vi "ADAM -12.vi"() -> ()   [LabVIEW 2016]
uses:
  <vilib>/Instr/_visa.llb/VISA Configure Serial Port (Instr).vi
panel:
  out "I 7_3":string
  out "I 6_3":string
  out "I 5_3":string
  out "I 4_3":string
  out "I 3_3":string
  out "I 2_3":string
  out "I 7_2":string
  out "I 6_2":string
  out "I 5_2":string
  out "I 4_2":string
  out "I 3_2":string
  out "I 2_2":string
  out "I 1_2":string
  out "I 0_2":string
  out "I 7_1":string
  out "I 6_1":string
  out "I 5_1":string
  out "I 4_1":string
  out "I 3_1":string
  out "I 2_1":string
  out "I 1_1":string
  out "I 0_1":string
  out "I 1_3":string
  out "I 0_3":string
  in  "rele 1_6":bool
  in  "rele 7_6":bool
  in  "rele 6_6":bool
  in  "rele 5_6":bool
  in  "rele 4_6":bool
  in  "rele 3_6":bool
  in  "rele 2_6":bool
  in  "rele 0_6":bool
  in  "rele 1_5":bool
  in  "rele 7_5":bool
  in  "rele 6_5":bool
  in  "rele 5_5":bool
  in  "rele 4_5":bool
  in  "rele 3_5":bool
  in  "rele 2_5":bool
  in  "rele 0_5":bool
  out "read buffer 3":string
  out "5_3":bool
  out "4_3":bool
  out "3_3":bool
  out "2_3":bool
  out "1_3":bool
  out "0_3":bool
  out "6_3":bool
  out "7_3":bool
  out "read buffer 2":string
  out "5_2":bool
  out "4_2":bool
  out "3_2":bool
  out "2_2":bool
  out "1_2":bool
  out "0_2":bool
  out "6_2":bool
  out "7_2":bool
  out "7_1":bool
  out "6_1":bool
  out "0_1":bool
  out "1_1":bool
  out "2_1":bool
  out "3_1":bool
  out "4_1":bool
  out "5_1":bool
  out "read buffer":string
  in  "all rele":bool
  in  "rele 1_4":bool
  in  "rele 7_4":bool
  in  "rele 6_4":bool
  in  "rele 5_4":bool
  in  "rele 4_4":bool
  in  "rele 3_4":bool
  in  "rele 2_4":bool
  in  "VISA rele":refnum<visa-resource-name>
  in  "rele 0_4":bool
  in  "stop":bool
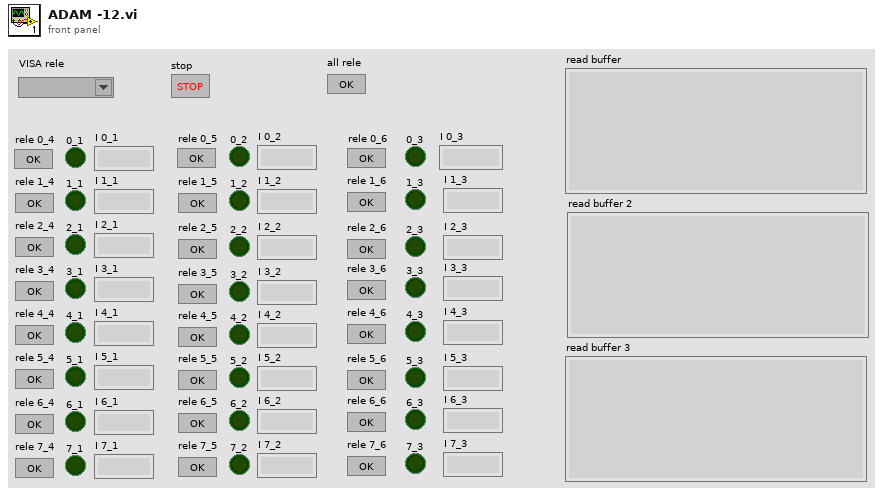
[diagram p1: front panel]
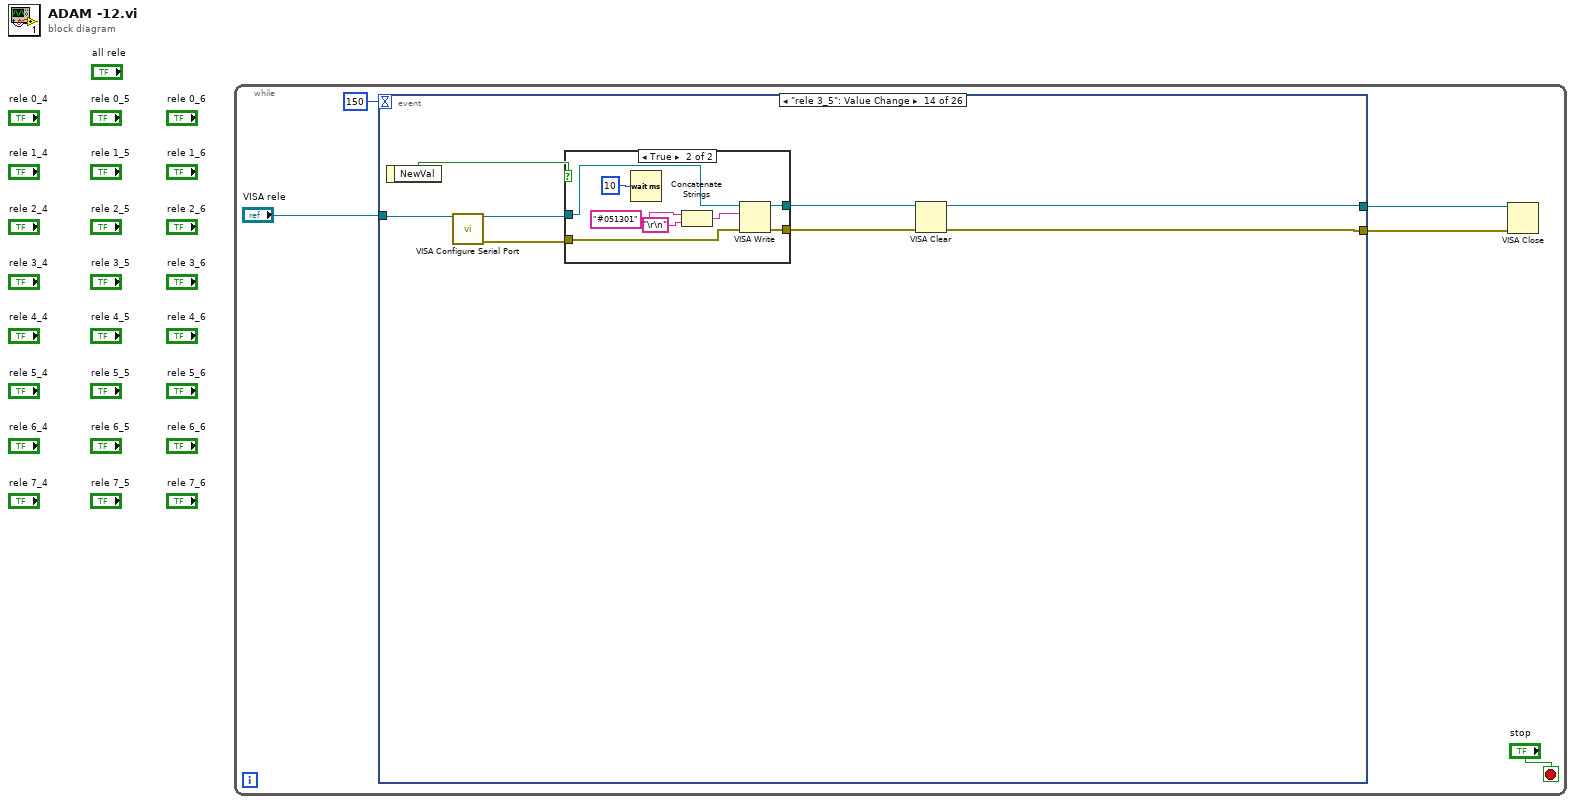
[diagram p0: block diagram]
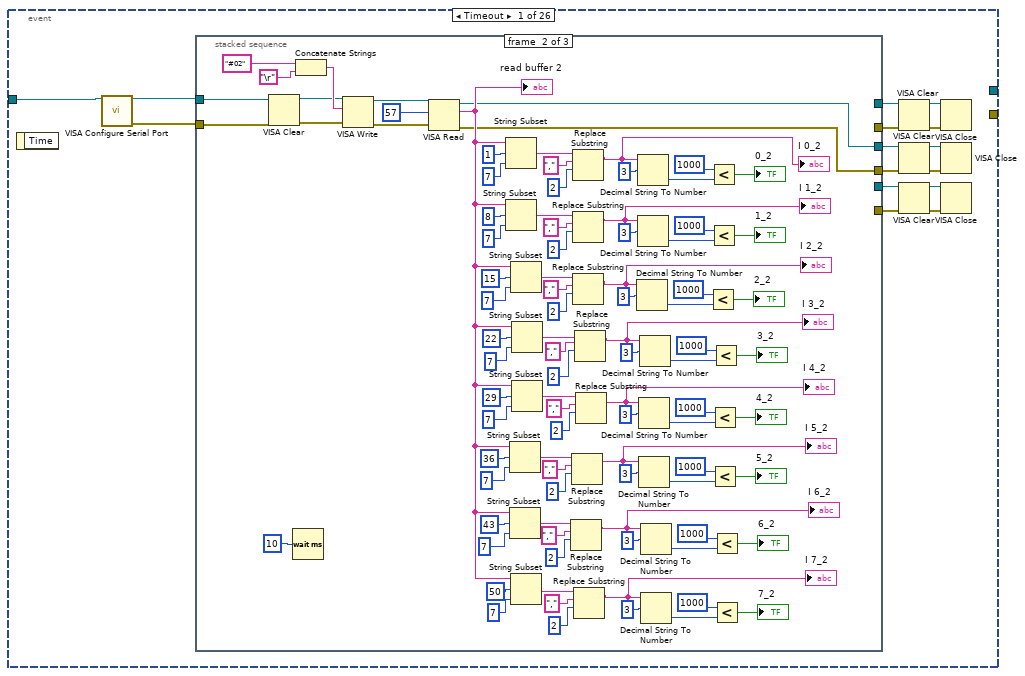
[diagram p2: hidden frame]
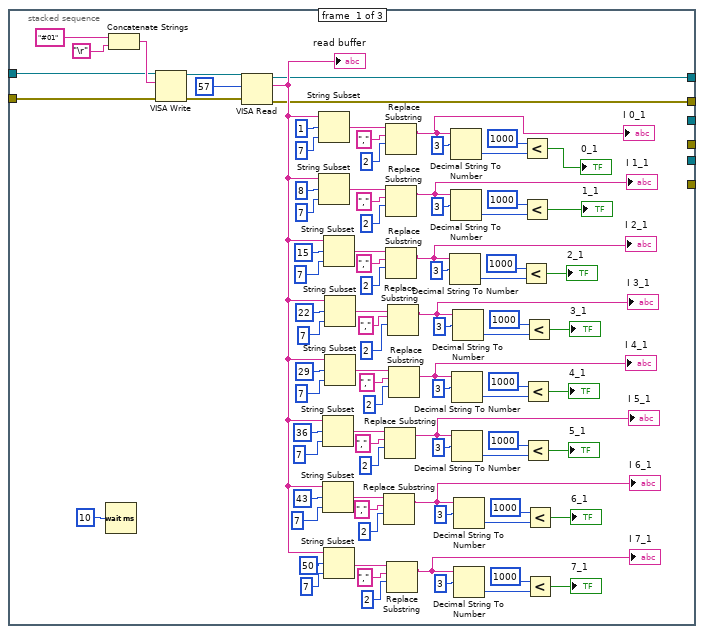
[diagram p3: hidden frame]
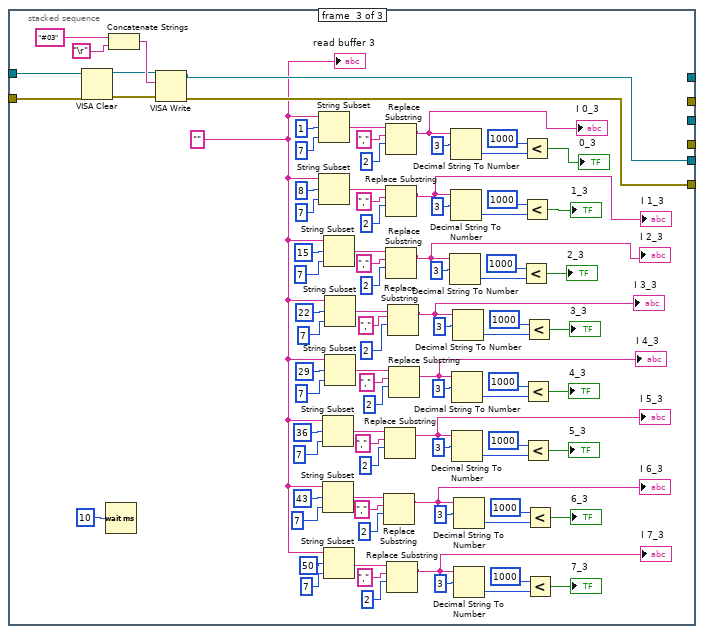
[diagram p4: hidden frame]
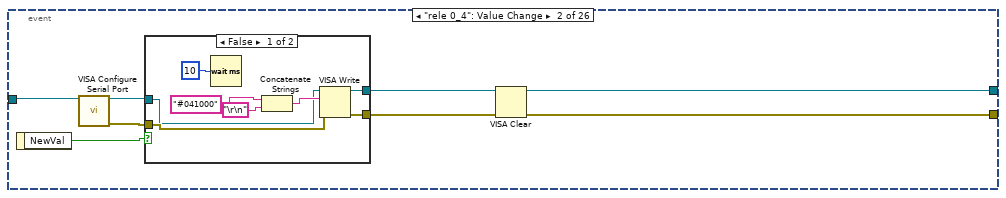
[diagram p5: hidden frame]
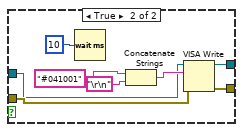
[diagram p6: hidden frame]
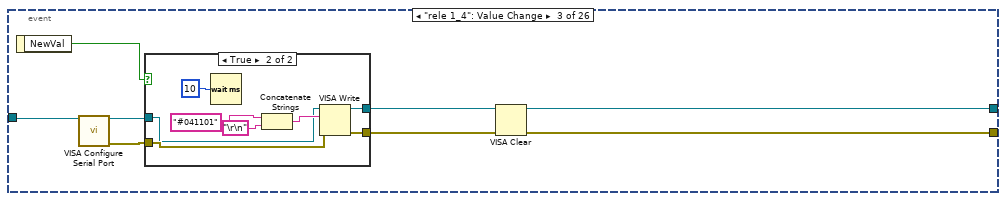
[diagram p7: hidden frame]
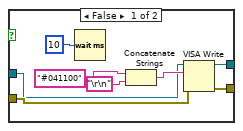
[diagram p8: hidden frame]
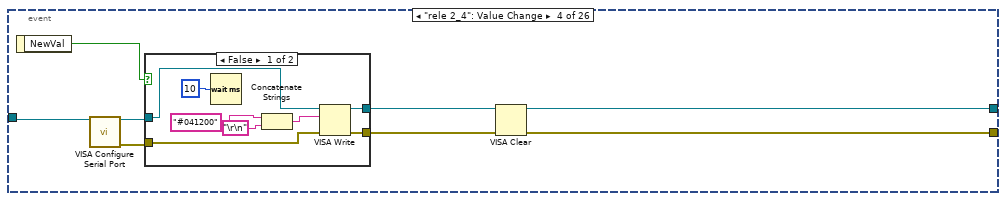
[diagram p9: hidden frame]
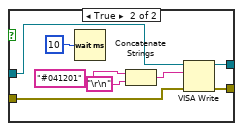
[diagram p10: hidden frame]
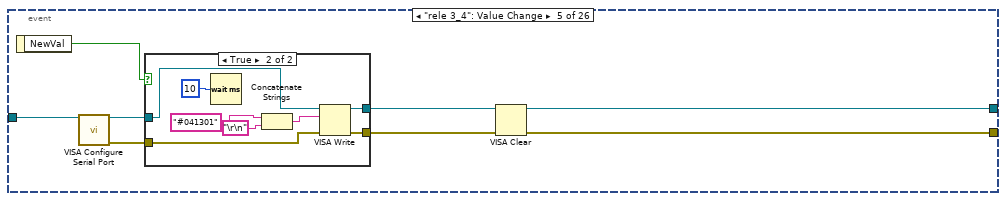
[diagram p11: hidden frame]
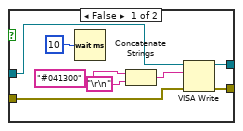
[diagram p12: hidden frame]
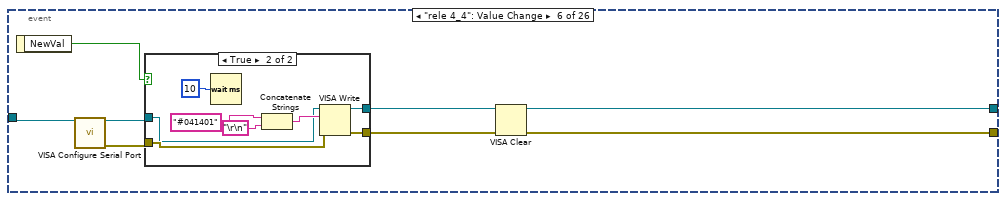
[diagram p13: hidden frame]
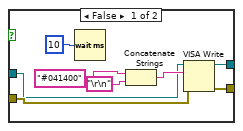
[diagram p14: hidden frame]
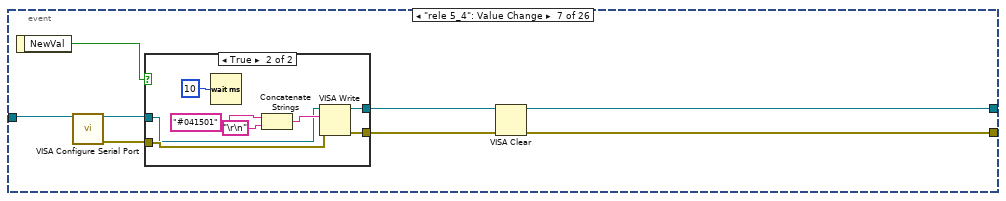
[diagram p15: hidden frame]
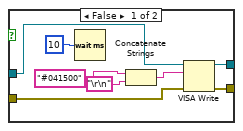
[diagram p16: hidden frame]
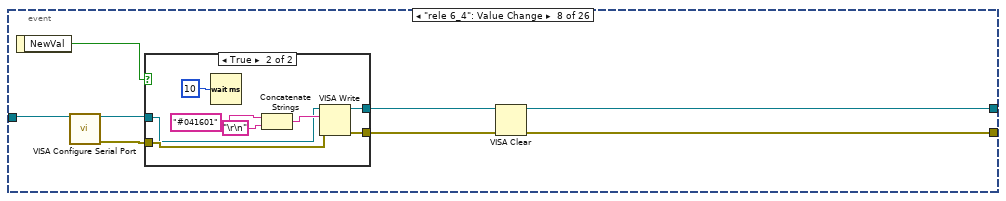
[diagram p17: hidden frame]
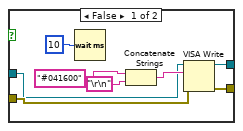
[diagram p18: hidden frame]
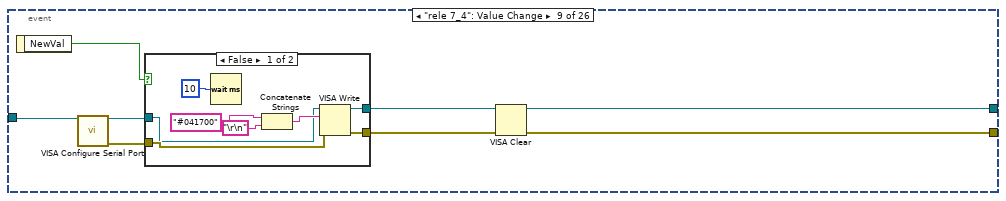
[diagram p19: hidden frame]
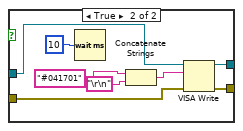
[diagram p20: hidden frame]
diagram:
  n1 = while {
    stop <- "stop" stop-if-true
    n2 = event shown="[13] \"rele 3_5\": Value Change" {
      selector: _ -> [_ _ _ _ _ _ _ _ _ _ _ _ _ _ _ _ _ _ _ _ _ _ _ _ _ _]
      dyn-events: _ -> [_ _ _ _ _ _ _ _ _ _ _ _ _ _ _ _ _ _ _ _ _ _ _ _ _ _]
      timeout: 150 -> [_ _ _ _ _ _ _ _ _ _ _ _ _ _ _ _ _ _ _ _ _ _ _ _ _ _]
      tunnel: "VISA rele" -> [w6 w298 w322 w346 w370 w394 w418 w442 w466 w490 w594 w618 w642 w666 w690 w714 w738 w762 w788 w810 w835 w858 w882 w906 w930 w954]
      tunnel: [_ w302 w326 w350 w374 w398 w422 w446 w470 w494 w598 w621 w646 w670 w694 w719 w742 w766 w790 w814 w838 w862 w886 w910 w934 w958] -> w3
      tunnel: [_ w301 w325 w349 w373 w397 w421 w445 w469 w493 w597 w622 w645 w669 w693 w718 w741 w765 w789 w813 w837 w861 w885 w909 w933 w957] -> w2
      event Timeout {
        n3 = event-data() -> ()  [unwired: 1 in, 1 out]
        n4 = call-poly "VISA Configure Serial Port"("VISA resource name"=w6) -> ("VISA resource name out"=w8:refnum<visa-resource-name>, "error out"=w7:errorcluster)  [unwired: 13 in]
        n5 = stacked-sequence {
          tunnel: w7 -> [w109 w124 w222]
          tunnel: w8 -> [w108 w123 w221]
          tunnel: [w62 _ _] -> w20
          tunnel: [w61 _ _] -> w17
          tunnel: [_ w126 _] -> w14
          tunnel: [_ w125 _] -> w13
          tunnel: [_ _ w218] -> w10
          tunnel: [_ _ w217] -> w9
          frame #0 {
            n6 = Wait (ms)(milliseconds to wait=u32 10) -> ()  [unwired: 1 out]
            n7 = Concatenate Strings("#01" ("string"), "\r") -> (w112:string)
            n8 = VISA Write(VISA resource name=w108, write buffer=w112, error in (no error)=w109) -> (VISA resource name out=w66:refnum<visa-resource-name>, error out=w65:errorcluster)  [unwired: 1 out]
            n9 = VISA Read(VISA resource name=w66, byte count=u32 57, error in (no error)=w65) -> (VISA resource name out=w61:refnum<visa-resource-name>, read buffer=w67:string, error out=w62:errorcluster)  [unwired: 1 out]
            "read buffer" <- w67
            n10 = String Subset(string=w67, offset (0)=1, length (rest)=7 ("length (rest)")) -> (substring=w84:string)
            n11 = String Subset(string=w67, offset (0)=8, length (rest)=7 ("length (rest)")) -> (substring=w89:string)
            n12 = String Subset(string=w67, offset (0)=36, length (rest)=7 ("length (rest)")) -> (substring=w101:string)
            n13 = String Subset(string=w67, offset (0)=43, length (rest)=7 ("length (rest)")) -> (substring=w104:string)
            n14 = String Subset(string=w67, offset (0)=15, length (rest)=7 ("length (rest)")) -> (substring=w92:string)
            n15 = String Subset(string=w67, offset (0)=50, length (rest)=7 ("length (rest)")) -> (substring=w107:string)
            n16 = String Subset(string=w67, offset (0)=22, length (rest)=7 ("length (rest)")) -> (substring=w95:string)
            n17 = String Subset(string=w67, offset (0)=29, length (rest)=7 ("length (rest)")) -> (substring=w98:string)
            n18 = Replace Substring(3:2 ("offset (0)"), 4:"," ("substring (\"\")"), 5:w104) -> (1:w22:string)  [unwired: 1 in, 1 out]
            "I 6_1" <- w22
            n19 = Replace Substring(3:2 ("offset (0)"), 4:"," ("substring (\"\")"), 5:w101) -> (1:w23:string)  [unwired: 1 in, 1 out]
            "I 5_1" <- w23
            n20 = Replace Substring(3:2 ("offset (0)"), 4:"," ("substring (\"\")"), 5:w84) -> (1:w28:string)  [unwired: 1 in, 1 out]
            "I 0_1" <- w28
            n21 = Replace Substring(3:2 ("offset (0)"), 4:"," ("substring (\"\")"), 5:w89) -> (1:w27:string)  [unwired: 1 in, 1 out]
            "I 1_1" <- w27
            n22 = Replace Substring(3:2 ("offset (0)"), 4:"," ("substring (\"\")"), 5:w92) -> (1:w26:string)  [unwired: 1 in, 1 out]
            "I 2_1" <- w26
            n23 = Replace Substring(3:2 ("offset (0)"), 4:"," ("substring (\"\")"), 5:w107) -> (1:w21:string)  [unwired: 1 in, 1 out]
            "I 7_1" <- w21
            n24 = Replace Substring(3:2 ("offset (0)"), 4:"," ("substring (\"\")"), 5:w95) -> (1:w25:string)  [unwired: 1 in, 1 out]
            "I 3_1" <- w25
            n25 = Replace Substring(3:2 ("offset (0)"), 4:"," ("substring (\"\")"), 5:w98) -> (1:w24:string)  [unwired: 1 in, 1 out]
            "I 4_1" <- w24
            n26 = Decimal String To Number(string=w26, offset=3) -> (number=w47:i32)  [unwired: 1 in, 1 out]
            n27 = Decimal String To Number(string=w28, offset=3) -> (number=w39:i32)  [unwired: 1 in, 1 out]
            n28 = Decimal String To Number(string=w27, offset=3) -> (number=w43:i32)  [unwired: 1 in, 1 out]
            n29 = Decimal String To Number(string=w24, offset=3) -> (number=w55:i32)  [unwired: 1 in, 1 out]
            n30 = Decimal String To Number(string=w23, offset=3) -> (number=w59:i32)  [unwired: 1 in, 1 out]
            n31 = Decimal String To Number(string=w25, offset=3) -> (number=w51:i32)  [unwired: 1 in, 1 out]
            n32 = Decimal String To Number(string=w22, offset=3) -> (number=w35:i32)  [unwired: 1 in, 1 out]
            n33 = Decimal String To Number(string=w21, offset=3) -> (number=w31:i32)  [unwired: 1 in, 1 out]
            n34 = Less?(x=1000, y=w47) -> (x < y?=→"2_1":bool)
            n35 = Less?(x=1000, y=w39) -> (x < y?=→"0_1":bool)
            n36 = Less?(x=1000, y=w43) -> (x < y?=→"1_1":bool)
            n37 = Less?(x=1000, y=w55) -> (x < y?=→"4_1":bool)
            n38 = Less?(x=1000, y=w59) -> (x < y?=→"5_1":bool)
            n39 = Less?(x=1000, y=w51) -> (x < y?=→"3_1":bool)
            n40 = Less?(x=1000, y=w35) -> (x < y?=→"6_1":bool)
            n41 = Less?(x=1000, y=w31) -> (x < y?=→"7_1":bool)
          }
          frame #1 {
            n42 = VISA Clear(VISA resource name=w123, error in (no error)=w124) -> (VISA resource name out=w121:refnum<visa-resource-name>, error out=w122:errorcluster)
            n43 = Wait (ms)(milliseconds to wait=u32 10) -> ()  [unwired: 1 out]
            n44 = Concatenate Strings("#02" ("string"), "\r") -> (w206:string)
            n45 = VISA Write(VISA resource name=w121, write buffer=w206, error in (no error)=w122) -> (VISA resource name out=w162:refnum<visa-resource-name>, error out=w161:errorcluster)  [unwired: 1 out]
            n46 = VISA Read(VISA resource name=w162, byte count=u32 57, error in (no error)=w161) -> (VISA resource name out=w125:refnum<visa-resource-name>, read buffer=w163:string, error out=w126:errorcluster)  [unwired: 1 out]
            "read buffer 2" <- w163
            n47 = String Subset(string=w163, offset (0)=1, length (rest)=7 ("length (rest)")) -> (substring=w180:string)
            n48 = String Subset(string=w163, offset (0)=8, length (rest)=7 ("length (rest)")) -> (substring=w185:string)
            n49 = String Subset(string=w163, offset (0)=36, length (rest)=7 ("length (rest)")) -> (substring=w197:string)
            n50 = String Subset(string=w163, offset (0)=43, length (rest)=7 ("length (rest)")) -> (substring=w200:string)
            n51 = String Subset(string=w163, offset (0)=15, length (rest)=7 ("length (rest)")) -> (substring=w188:string)
            n52 = String Subset(string=w163, offset (0)=50, length (rest)=7 ("length (rest)")) -> (substring=w203:string)
            n53 = String Subset(string=w163, offset (0)=22, length (rest)=7 ("length (rest)")) -> (substring=w191:string)
            n54 = String Subset(string=w163, offset (0)=29, length (rest)=7 ("length (rest)")) -> (substring=w194:string)
            n55 = Replace Substring(3:2 ("offset (0)"), 4:"," ("substring (\"\")"), 5:w200) -> (1:w114:string)  [unwired: 1 in, 1 out]
            "I 6_2" <- w114
            n56 = Replace Substring(3:2 ("offset (0)"), 4:"," ("substring (\"\")"), 5:w197) -> (1:w115:string)  [unwired: 1 in, 1 out]
            "I 5_2" <- w115
            n57 = Replace Substring(3:2 ("offset (0)"), 4:"," ("substring (\"\")"), 5:w180) -> (1:w120:string)  [unwired: 1 in, 1 out]
            "I 0_2" <- w120
            n58 = Replace Substring(3:2 ("offset (0)"), 4:"," ("substring (\"\")"), 5:w185) -> (1:w119:string)  [unwired: 1 in, 1 out]
            "I 1_2" <- w119
            n59 = Replace Substring(3:2 ("offset (0)"), 4:"," ("substring (\"\")"), 5:w188) -> (1:w118:string)  [unwired: 1 in, 1 out]
            "I 2_2" <- w118
            n60 = Replace Substring(3:2 ("offset (0)"), 4:"," ("substring (\"\")"), 5:w203) -> (1:w113:string)  [unwired: 1 in, 1 out]
            "I 7_2" <- w113
            n61 = Replace Substring(3:2 ("offset (0)"), 4:"," ("substring (\"\")"), 5:w191) -> (1:w117:string)  [unwired: 1 in, 1 out]
            "I 3_2" <- w117
            n62 = Replace Substring(3:2 ("offset (0)"), 4:"," ("substring (\"\")"), 5:w194) -> (1:w116:string)  [unwired: 1 in, 1 out]
            "I 4_2" <- w116
            n63 = Decimal String To Number(string=w118, offset=3) -> (number=w145:i32)  [unwired: 1 in, 1 out]
            n64 = Decimal String To Number(string=w120, offset=3) -> (number=w137:i32)  [unwired: 1 in, 1 out]
            n65 = Decimal String To Number(string=w119, offset=3) -> (number=w141:i32)  [unwired: 1 in, 1 out]
            n66 = Decimal String To Number(string=w116, offset=3) -> (number=w153:i32)  [unwired: 1 in, 1 out]
            n67 = Decimal String To Number(string=w115, offset=3) -> (number=w157:i32)  [unwired: 1 in, 1 out]
            n68 = Decimal String To Number(string=w117, offset=3) -> (number=w149:i32)  [unwired: 1 in, 1 out]
            n69 = Decimal String To Number(string=w114, offset=3) -> (number=w133:i32)  [unwired: 1 in, 1 out]
            n70 = Decimal String To Number(string=w113, offset=3) -> (number=w129:i32)  [unwired: 1 in, 1 out]
            n71 = Less?(x=1000, y=w145) -> (x < y?=→"2_2":bool)
            n72 = Less?(x=1000, y=w137) -> (x < y?=→"0_2":bool)
            n73 = Less?(x=1000, y=w141) -> (x < y?=→"1_2":bool)
            n74 = Less?(x=1000, y=w153) -> (x < y?=→"4_2":bool)
            n75 = Less?(x=1000, y=w157) -> (x < y?=→"5_2":bool)
            n76 = Less?(x=1000, y=w149) -> (x < y?=→"3_2":bool)
            n77 = Less?(x=1000, y=w133) -> (x < y?=→"6_2":bool)
            n78 = Less?(x=1000, y=w129) -> (x < y?=→"7_2":bool)
          }
          frame #2 {
            w216 = "" ("string")
            n79 = VISA Clear(VISA resource name=w221, error in (no error)=w222) -> (VISA resource name out=w219:refnum<visa-resource-name>, error out=w220:errorcluster)
            n80 = Wait (ms)(milliseconds to wait=u32 10) -> ()  [unwired: 1 out]
            n81 = Concatenate Strings("#03" ("string"), "\r") -> (w297:string)
            n82 = VISA Write(VISA resource name=w219, write buffer=w297, error in (no error)=w220) -> (VISA resource name out=w218:refnum<visa-resource-name>, error out=w217:errorcluster)  [unwired: 1 out]
            n83 = String Subset(string=w216, offset (0)=1, length (rest)=7 ("length (rest)")) -> (substring=w214:string)
            n84 = String Subset(string=w216, offset (0)=8, length (rest)=7 ("length (rest)")) -> (substring=w276:string)
            n85 = String Subset(string=w216, offset (0)=36, length (rest)=7 ("length (rest)")) -> (substring=w288:string)
            n86 = String Subset(string=w216, offset (0)=43, length (rest)=7 ("length (rest)")) -> (substring=w291:string)
            n87 = String Subset(string=w216, offset (0)=15, length (rest)=7 ("length (rest)")) -> (substring=w279:string)
            n88 = String Subset(string=w216, offset (0)=50, length (rest)=7 ("length (rest)")) -> (substring=w294:string)
            n89 = String Subset(string=w216, offset (0)=22, length (rest)=7 ("length (rest)")) -> (substring=w282:string)
            n90 = String Subset(string=w216, offset (0)=29, length (rest)=7 ("length (rest)")) -> (substring=w285:string)
            n91 = Replace Substring(3:2 ("offset (0)"), 4:"," ("substring (\"\")"), 5:w291) -> (1:w208:string)  [unwired: 1 in, 1 out]
            "I 6_3" <- w208
            n92 = Replace Substring(3:2 ("offset (0)"), 4:"," ("substring (\"\")"), 5:w288) -> (1:w209:string)  [unwired: 1 in, 1 out]
            "I 5_3" <- w209
            n93 = Replace Substring(3:2 ("offset (0)"), 4:"," ("substring (\"\")"), 5:w214) -> (1:w213:string)  [unwired: 1 in, 1 out]
            "I 0_3" <- w213
            n94 = Replace Substring(3:2 ("offset (0)"), 4:"," ("substring (\"\")"), 5:w276) -> (1:w215:string)  [unwired: 1 in, 1 out]
            "I 1_3" <- w215
            n95 = Replace Substring(3:2 ("offset (0)"), 4:"," ("substring (\"\")"), 5:w279) -> (1:w212:string)  [unwired: 1 in, 1 out]
            "I 2_3" <- w212
            n96 = Replace Substring(3:2 ("offset (0)"), 4:"," ("substring (\"\")"), 5:w294) -> (1:w207:string)  [unwired: 1 in, 1 out]
            "I 7_3" <- w207
            n97 = Replace Substring(3:2 ("offset (0)"), 4:"," ("substring (\"\")"), 5:w282) -> (1:w211:string)  [unwired: 1 in, 1 out]
            "I 3_3" <- w211
            n98 = Replace Substring(3:2 ("offset (0)"), 4:"," ("substring (\"\")"), 5:w285) -> (1:w210:string)  [unwired: 1 in, 1 out]
            "I 4_3" <- w210
            n99 = Decimal String To Number(string=w212, offset=3) -> (number=w241:i32)  [unwired: 1 in, 1 out]
            n100 = Decimal String To Number(string=w213, offset=3) -> (number=w233:i32)  [unwired: 1 in, 1 out]
            n101 = Decimal String To Number(string=w215, offset=3) -> (number=w237:i32)  [unwired: 1 in, 1 out]
            n102 = Decimal String To Number(string=w210, offset=3) -> (number=w249:i32)  [unwired: 1 in, 1 out]
            n103 = Decimal String To Number(string=w209, offset=3) -> (number=w253:i32)  [unwired: 1 in, 1 out]
            n104 = Decimal String To Number(string=w211, offset=3) -> (number=w245:i32)  [unwired: 1 in, 1 out]
            n105 = Decimal String To Number(string=w208, offset=3) -> (number=w229:i32)  [unwired: 1 in, 1 out]
            n106 = Decimal String To Number(string=w207, offset=3) -> (number=w225:i32)  [unwired: 1 in, 1 out]
            n107 = Less?(x=1000, y=w241) -> (x < y?=→"2_3":bool)
            n108 = Less?(x=1000, y=w233) -> (x < y?=→"0_3":bool)
            n109 = Less?(x=1000, y=w237) -> (x < y?=→"1_3":bool)
            n110 = Less?(x=1000, y=w249) -> (x < y?=→"4_3":bool)
            n111 = Less?(x=1000, y=w253) -> (x < y?=→"5_3":bool)
            n112 = Less?(x=1000, y=w245) -> (x < y?=→"3_3":bool)
            n113 = Less?(x=1000, y=w229) -> (x < y?=→"6_3":bool)
            n114 = Less?(x=1000, y=w225) -> (x < y?=→"7_3":bool)
            "read buffer 3" <- w216
          }
        }
        n115 = VISA Clear(VISA resource name=w17, error in (no error)=w20) -> (VISA resource name out=w15:refnum<visa-resource-name>, error out=w16:errorcluster)
        n116 = VISA Clear(VISA resource name=w13, error in (no error)=w14) -> (VISA resource name out=w19:refnum<visa-resource-name>, error out=w18:errorcluster)
        n117 = VISA Clear(VISA resource name=w10, error in (no error)=w9) -> (VISA resource name out=w12:refnum<visa-resource-name>, error out=w11:errorcluster)
        n118 = VISA Close(VISA resource name=w15, error in (no error)=w16) -> ()  [unwired: 1 out]
        n119 = VISA Close(VISA resource name=w19, error in (no error)=w18) -> ()  [unwired: 1 out]
        n120 = VISA Close(VISA resource name=w12, error in (no error)=w11) -> ()  [unwired: 1 out]
      }
      event "rele 0_4": Value Change {
        n121 = event-data() -> ("NewVal"=w305:bool)  [unwired: 1 in]
        n122 = call-poly "VISA Configure Serial Port"("VISA resource name"=w298) -> ("VISA resource name out"=w299:refnum<visa-resource-name>, "error out"=w300:errorcluster)  [unwired: 13 in]
        n123 = case shown="False" w305 {
          tunnel: [w310 w318] -> w303
          tunnel: [w309 w317] -> w304
          tunnel: w300 -> [w308 w316]
          tunnel: w299 -> [w307 w315]
          frame False {
            n124 = Wait (ms)(milliseconds to wait=u32 10) -> ()  [unwired: 1 out]
            n125 = Concatenate Strings("#041000" ("string"), "\r\n") -> (w313:string)
            n126 = VISA Write(VISA resource name=w307, write buffer=w313, error in (no error)=w308) -> (VISA resource name out=w310:refnum<visa-resource-name>, error out=w309:errorcluster)  [unwired: 1 out]
          }
          frame True {
            n127 = Wait (ms)(milliseconds to wait=u32 10) -> ()  [unwired: 1 out]
            n128 = Concatenate Strings("#041001" ("string"), "\r\n") -> (w321:string)
            n129 = VISA Write(VISA resource name=w315, write buffer=w321, error in (no error)=w316) -> (VISA resource name out=w318:refnum<visa-resource-name>, error out=w317:errorcluster)  [unwired: 1 out]
          }
        }
        n130 = VISA Clear(VISA resource name=w303, error in (no error)=w304) -> (VISA resource name out=w301:refnum<visa-resource-name>, error out=w302:errorcluster)
      }
      event "rele 1_4": Value Change {
        n131 = event-data() -> ("NewVal"=w329:bool)  [unwired: 1 in]
        n132 = call-poly "VISA Configure Serial Port"("VISA resource name"=w322) -> ("VISA resource name out"=w324:refnum<visa-resource-name>, "error out"=w323:errorcluster)  [unwired: 13 in]
        n133 = case shown="True" w329 {
          tunnel: [w334 w342] -> w328
          tunnel: [w333 w341] -> w327
          tunnel: w323 -> [w331 w339]
          tunnel: w324 -> [w330 w338]
          frame False {
            n134 = Wait (ms)(milliseconds to wait=u32 10) -> ()  [unwired: 1 out]
            n135 = Concatenate Strings("#041100" ("string"), "\r\n") -> (w337:string)
            n136 = VISA Write(VISA resource name=w330, write buffer=w337, error in (no error)=w331) -> (VISA resource name out=w333:refnum<visa-resource-name>, error out=w334:errorcluster)  [unwired: 1 out]
          }
          frame True {
            n137 = Wait (ms)(milliseconds to wait=u32 10) -> ()  [unwired: 1 out]
            n138 = Concatenate Strings("#041101" ("string"), "\r\n") -> (w345:string)
            n139 = VISA Write(VISA resource name=w338, write buffer=w345, error in (no error)=w339) -> (VISA resource name out=w341:refnum<visa-resource-name>, error out=w342:errorcluster)  [unwired: 1 out]
          }
        }
        n140 = VISA Clear(VISA resource name=w327, error in (no error)=w328) -> (VISA resource name out=w325:refnum<visa-resource-name>, error out=w326:errorcluster)
      }
      event "rele 2_4": Value Change {
        n141 = event-data() -> ("NewVal"=w353:bool)  [unwired: 1 in]
        n142 = call-poly "VISA Configure Serial Port"("VISA resource name"=w346) -> ("VISA resource name out"=w348:refnum<visa-resource-name>, "error out"=w347:errorcluster)  [unwired: 13 in]
        n143 = case shown="False" w353 {
          tunnel: [w356 w366] -> w352
          tunnel: [w355 w365] -> w351
          tunnel: w348 -> [w358 w364]
          tunnel: w347 -> [w357 w363]
          frame False {
            n144 = Wait (ms)(milliseconds to wait=u32 10) -> ()  [unwired: 1 out]
            n145 = Concatenate Strings("#041200" ("string"), "\r\n") -> (w361:string)
            n146 = VISA Write(VISA resource name=w358, write buffer=w361, error in (no error)=w357) -> (VISA resource name out=w355:refnum<visa-resource-name>, error out=w356:errorcluster)  [unwired: 1 out]
          }
          frame True {
            n147 = Wait (ms)(milliseconds to wait=u32 10) -> ()  [unwired: 1 out]
            n148 = Concatenate Strings("#041201" ("string"), "\r\n") -> (w369:string)
            n149 = VISA Write(VISA resource name=w364, write buffer=w369, error in (no error)=w363) -> (VISA resource name out=w365:refnum<visa-resource-name>, error out=w366:errorcluster)  [unwired: 1 out]
          }
        }
        n150 = VISA Clear(VISA resource name=w351, error in (no error)=w352) -> (VISA resource name out=w349:refnum<visa-resource-name>, error out=w350:errorcluster)
      }
      event "rele 3_4": Value Change {
        n151 = event-data() -> ("NewVal"=w377:bool)  [unwired: 1 in]
        n152 = call-poly "VISA Configure Serial Port"("VISA resource name"=w370) -> ("VISA resource name out"=w372:refnum<visa-resource-name>, "error out"=w371:errorcluster)  [unwired: 13 in]
        n153 = case shown="True" w377 {
          tunnel: w372 -> [w382 w390]
          tunnel: w371 -> [w381 w389]
          tunnel: [w380 w387] -> w376
          tunnel: [w379 w388] -> w375
          frame False {
            n154 = Wait (ms)(milliseconds to wait=u32 10) -> ()  [unwired: 1 out]
            n155 = Concatenate Strings("#041300" ("string"), "\r\n") -> (w385:string)
            n156 = VISA Write(VISA resource name=w382, write buffer=w385, error in (no error)=w381) -> (VISA resource name out=w379:refnum<visa-resource-name>, error out=w380:errorcluster)  [unwired: 1 out]
          }
          frame True {
            n157 = Wait (ms)(milliseconds to wait=u32 10) -> ()  [unwired: 1 out]
            n158 = Concatenate Strings("#041301" ("string"), "\r\n") -> (w393:string)
            n159 = VISA Write(VISA resource name=w390, write buffer=w393, error in (no error)=w389) -> (VISA resource name out=w388:refnum<visa-resource-name>, error out=w387:errorcluster)  [unwired: 1 out]
          }
        }
        n160 = VISA Clear(VISA resource name=w375, error in (no error)=w376) -> (VISA resource name out=w373:refnum<visa-resource-name>, error out=w374:errorcluster)
      }
      event "rele 4_4": Value Change {
        n161 = event-data() -> ("NewVal"=w401:bool)  [unwired: 1 in]
        n162 = call-poly "VISA Configure Serial Port"("VISA resource name"=w394) -> ("VISA resource name out"=w395:refnum<visa-resource-name>, "error out"=w396:errorcluster)  [unwired: 13 in]
        n163 = case shown="True" w401 {
          tunnel: [w404 w414] -> w400
          tunnel: [w403 w413] -> w399
          tunnel: w396 -> [w406 w412]
          tunnel: w395 -> [w405 w411]
          frame False {
            n164 = Wait (ms)(milliseconds to wait=u32 10) -> ()  [unwired: 1 out]
            n165 = Concatenate Strings("#041400" ("string"), "\r\n") -> (w409:string)
            n166 = VISA Write(VISA resource name=w405, write buffer=w409, error in (no error)=w406) -> (VISA resource name out=w403:refnum<visa-resource-name>, error out=w404:errorcluster)  [unwired: 1 out]
          }
          frame True {
            n167 = Wait (ms)(milliseconds to wait=u32 10) -> ()  [unwired: 1 out]
            n168 = Concatenate Strings("#041401" ("string"), "\r\n") -> (w417:string)
            n169 = VISA Write(VISA resource name=w411, write buffer=w417, error in (no error)=w412) -> (VISA resource name out=w413:refnum<visa-resource-name>, error out=w414:errorcluster)  [unwired: 1 out]
          }
        }
        n170 = VISA Clear(VISA resource name=w399, error in (no error)=w400) -> (VISA resource name out=w397:refnum<visa-resource-name>, error out=w398:errorcluster)
      }
      event "rele 5_4": Value Change {
        n171 = event-data() -> ("NewVal"=w425:bool)  [unwired: 1 in]
        n172 = call-poly "VISA Configure Serial Port"("VISA resource name"=w418) -> ("VISA resource name out"=w420:refnum<visa-resource-name>, "error out"=w419:errorcluster)  [unwired: 13 in]
        n173 = case shown="True" w425 {
          tunnel: [w429 w437] -> w424
          tunnel: [w428 w436] -> w423
          tunnel: w420 -> [w427 w434]
          tunnel: w419 -> [w426 w435]
          frame False {
            n174 = Wait (ms)(milliseconds to wait=u32 10) -> ()  [unwired: 1 out]
            n175 = Concatenate Strings("#041500" ("string"), "\r\n") -> (w433:string)
            n176 = VISA Write(VISA resource name=w427, write buffer=w433, error in (no error)=w426) -> (VISA resource name out=w428:refnum<visa-resource-name>, error out=w429:errorcluster)  [unwired: 1 out]
          }
          frame True {
            n177 = Wait (ms)(milliseconds to wait=u32 10) -> ()  [unwired: 1 out]
            n178 = Concatenate Strings("#041501" ("string"), "\r\n") -> (w441:string)
            n179 = VISA Write(VISA resource name=w434, write buffer=w441, error in (no error)=w435) -> (VISA resource name out=w436:refnum<visa-resource-name>, error out=w437:errorcluster)  [unwired: 1 out]
          }
        }
        n180 = VISA Clear(VISA resource name=w423, error in (no error)=w424) -> (VISA resource name out=w421:refnum<visa-resource-name>, error out=w422:errorcluster)
      }
      event "rele 6_4": Value Change {
        n181 = event-data() -> ("NewVal"=w449:bool)  [unwired: 1 in]
        n182 = call-poly "VISA Configure Serial Port"("VISA resource name"=w442) -> ("VISA resource name out"=w444:refnum<visa-resource-name>, "error out"=w443:errorcluster)  [unwired: 13 in]
        n183 = case shown="True" w449 {
          tunnel: [w454 w461] -> w448
          tunnel: [w453 w462] -> w447
          tunnel: w443 -> [w452 w460]
          tunnel: w444 -> [w451 w459]
          frame False {
            n184 = Wait (ms)(milliseconds to wait=u32 10) -> ()  [unwired: 1 out]
            n185 = Concatenate Strings("#041600" ("string"), "\r\n") -> (w457:string)
            n186 = VISA Write(VISA resource name=w451, write buffer=w457, error in (no error)=w452) -> (VISA resource name out=w453:refnum<visa-resource-name>, error out=w454:errorcluster)  [unwired: 1 out]
          }
          frame True {
            n187 = Wait (ms)(milliseconds to wait=u32 10) -> ()  [unwired: 1 out]
            n188 = Concatenate Strings("#041601" ("string"), "\r\n") -> (w465:string)
            n189 = VISA Write(VISA resource name=w459, write buffer=w465, error in (no error)=w460) -> (VISA resource name out=w462:refnum<visa-resource-name>, error out=w461:errorcluster)  [unwired: 1 out]
          }
        }
        n190 = VISA Clear(VISA resource name=w447, error in (no error)=w448) -> (VISA resource name out=w445:refnum<visa-resource-name>, error out=w446:errorcluster)
      }
      event "rele 7_4": Value Change {
        n191 = event-data() -> ("NewVal"=w473:bool)  [unwired: 1 in]
        n192 = call-poly "VISA Configure Serial Port"("VISA resource name"=w466) -> ("VISA resource name out"=w468:refnum<visa-resource-name>, "error out"=w467:errorcluster)  [unwired: 13 in]
        n193 = case shown="False" w473 {
          tunnel: w467 -> [w477 w482]
          tunnel: w468 -> [w476 w483]
          tunnel: [w475 w486] -> w472
          tunnel: [w474 w485] -> w471
          frame False {
            n194 = Wait (ms)(milliseconds to wait=u32 10) -> ()  [unwired: 1 out]
            n195 = Concatenate Strings("#041700" ("string"), "\r\n") -> (w481:string)
            n196 = VISA Write(VISA resource name=w476, write buffer=w481, error in (no error)=w477) -> (VISA resource name out=w474:refnum<visa-resource-name>, error out=w475:errorcluster)  [unwired: 1 out]
          }
          frame True {
            n197 = Wait (ms)(milliseconds to wait=u32 10) -> ()  [unwired: 1 out]
            n198 = Concatenate Strings("#041701" ("string"), "\r\n") -> (w489:string)
            n199 = VISA Write(VISA resource name=w483, write buffer=w489, error in (no error)=w482) -> (VISA resource name out=w485:refnum<visa-resource-name>, error out=w486:errorcluster)  [unwired: 1 out]
          }
        }
        n200 = VISA Clear(VISA resource name=w471, error in (no error)=w472) -> (VISA resource name out=w469:refnum<visa-resource-name>, error out=w470:errorcluster)
      }
      event "all rele": Value Change {
        n201 = event-data() -> ("NewVal"=w497:bool)  [unwired: 1 in]
        n202 = call-poly "VISA Configure Serial Port"("VISA resource name"=w490) -> ("VISA resource name out"=w491:refnum<visa-resource-name>, "error out"=w492:errorcluster)  [unwired: 13 in]
        n203 = case shown="True" w497 {
          selector: w497 -> [w498 w546]
          tunnel: w492 -> [w502 w550]
          tunnel: w491 -> [w501 w549]
          tunnel: [w500 w548] -> w496
          tunnel: [w499 w547] -> w495
          frame False {
            n204 = stacked-sequence {
              tunnel: w502 -> [w509 w524 w537]
              tunnel: w501 -> [w508 w523 w536]
              tunnel: [_ _ w534] -> w500
              tunnel: [_ _ w533] -> w499
              frame #0 {
                n205 = flat-sequence {
                  tunnel: w509 -> [w513]
                  tunnel: w508 -> [w512]
                  tunnel: [w511] -> w505
                  tunnel: [w510] -> w504
                  frame #0 {
                    n206 = Wait (ms)(milliseconds to wait=u32 20) -> ()  [unwired: 1 out]
                    n207 = Concatenate Strings("#060000" ("string"), "\r\n") -> (w517:string)
                    n208 = VISA Write(VISA resource name=w512, write buffer=w517, error in (no error)=w513) -> (VISA resource name out=w510:refnum<visa-resource-name>, error out=w511:errorcluster)  [unwired: 1 out]
                  }
                }
                n209 = VISA Clear(VISA resource name=w504, error in (no error)=w505) -> (VISA resource name out=w506:refnum<visa-resource-name>, error out=w507:errorcluster)
                n210 = VISA Close(VISA resource name=w506, error in (no error)=w507) -> ()  [unwired: 1 out]
                n211 = Wait (ms)(milliseconds to wait=u32 20) -> ()  [unwired: 1 out]
              }
              frame #1 {
                n212 = flat-sequence {
                  tunnel: w524 -> [w528]
                  tunnel: w523 -> [w527]
                  tunnel: [w526] -> w520
                  tunnel: [w525] -> w519
                  frame #0 {
                    n213 = Wait (ms)(milliseconds to wait=u32 20) -> ()  [unwired: 1 out]
                    n214 = Concatenate Strings("#050000" ("string"), "\r\n") -> (w532:string)
                    n215 = VISA Write(VISA resource name=w527, write buffer=w532, error in (no error)=w528) -> (VISA resource name out=w525:refnum<visa-resource-name>, error out=w526:errorcluster)  [unwired: 1 out]
                  }
                }
                n216 = VISA Clear(VISA resource name=w519, error in (no error)=w520) -> (VISA resource name out=w521:refnum<visa-resource-name>, error out=w522:errorcluster)
                n217 = VISA Close(VISA resource name=w521, error in (no error)=w522) -> ()  [unwired: 1 out]
                n218 = Wait (ms)(milliseconds to wait=u32 20) -> ()  [unwired: 1 out]
              }
              frame #2 {
                n219 = flat-sequence {
                  tunnel: w537 -> [w545]
                  tunnel: w536 -> [w544]
                  tunnel: [w539] -> w534
                  tunnel: [w538] -> w533
                  frame #0 {
                    n220 = Wait (ms)(milliseconds to wait=u32 20) -> ()  [unwired: 1 out]
                    n221 = Concatenate Strings("#040000" ("string"), "\r\n") -> (w543:string)
                    n222 = VISA Write(VISA resource name=w544, write buffer=w543, error in (no error)=w545) -> (VISA resource name out=w538:refnum<visa-resource-name>, error out=w539:errorcluster)  [unwired: 1 out]
                  }
                }
                n223 = Wait (ms)(milliseconds to wait=u32 20) -> ()  [unwired: 1 out]
              }
            }
            n224 = local write "rele 0_4"(w498) -> ()
            n225 = local write "rele 1_4"(w498) -> ()
            n226 = local write "rele 2_4"(w498) -> ()
            n227 = local write "rele 3_4"(w498) -> ()
            n228 = local write "rele 4_4"(w498) -> ()
            n229 = local write "rele 5_4"(w498) -> ()
            n230 = local write "rele 6_4"(w498) -> ()
            n231 = local write "rele 7_4"(w498) -> ()
            n232 = local write "rele 0_5"(w498) -> ()
            n233 = local write "rele 1_5"(w498) -> ()
            n234 = local write "rele 2_5"(w498) -> ()
            n235 = local write "rele 3_5"(w498) -> ()
            n236 = local write "rele 4_5"(w498) -> ()
            n237 = local write "rele 5_5"(w498) -> ()
            n238 = local write "rele 6_5"(w498) -> ()
            n239 = local write "rele 7_5"(w498) -> ()
            n240 = local write "rele 0_6"(w498) -> ()
            n241 = local write "rele 1_6"(w498) -> ()
            n242 = local write "rele 2_6"(w498) -> ()
            n243 = local write "rele 3_6"(w498) -> ()
            n244 = local write "rele 4_6"(w498) -> ()
            n245 = local write "rele 5_6"(w498) -> ()
            n246 = local write "rele 6_6"(w498) -> ()
            n247 = local write "rele 7_6"(w498) -> ()
          }
          frame True {
            n248 = stacked-sequence {
              tunnel: w550 -> [w557 w572 w584]
              tunnel: w549 -> [w556 w571 w585]
              tunnel: [_ _ w582] -> w548
              tunnel: [_ _ w581] -> w547
              frame #0 {
                n249 = flat-sequence {
                  tunnel: w557 -> [w562]
                  tunnel: w556 -> [w561]
                  tunnel: [w559] -> w554
                  tunnel: [w558] -> w553
                  frame #0 {
                    n250 = Wait (ms)(milliseconds to wait=u32 20) -> ()  [unwired: 1 out]
                    n251 = Concatenate Strings("#0400FF" ("string"), "\r\n") -> (w565:string)
                    n252 = VISA Write(VISA resource name=w561, write buffer=w565, error in (no error)=w562) -> (VISA resource name out=w558:refnum<visa-resource-name>, error out=w559:errorcluster)  [unwired: 1 out]
                  }
                }
                n253 = VISA Clear(VISA resource name=w553, error in (no error)=w554) -> (VISA resource name out=w552:refnum<visa-resource-name>, error out=w555:errorcluster)
                n254 = VISA Close(VISA resource name=w552, error in (no error)=w555) -> ()  [unwired: 1 out]
                n255 = Wait (ms)(milliseconds to wait=u32 20) -> ()  [unwired: 1 out]
              }
              frame #1 {
                n256 = flat-sequence {
                  tunnel: w572 -> [w577]
                  tunnel: w571 -> [w576]
                  tunnel: [w574] -> w569
                  tunnel: [w573] -> w568
                  frame #0 {
                    n257 = Wait (ms)(milliseconds to wait=u32 20) -> ()  [unwired: 1 out]
                    n258 = Concatenate Strings("#0500FF" ("string"), "\r\n") -> (w580:string)
                    n259 = VISA Write(VISA resource name=w576, write buffer=w580, error in (no error)=w577) -> (VISA resource name out=w573:refnum<visa-resource-name>, error out=w574:errorcluster)  [unwired: 1 out]
                  }
                }
                n260 = VISA Clear(VISA resource name=w568, error in (no error)=w569) -> (VISA resource name out=w567:refnum<visa-resource-name>, error out=w570:errorcluster)
                n261 = VISA Close(VISA resource name=w567, error in (no error)=w570) -> ()  [unwired: 1 out]
                n262 = Wait (ms)(milliseconds to wait=u32 20) -> ()  [unwired: 1 out]
              }
              frame #2 {
                n263 = flat-sequence {
                  tunnel: w585 -> [w589]
                  tunnel: w584 -> [w588]
                  tunnel: [w587] -> w582
                  tunnel: [w586] -> w581
                  frame #0 {
                    n264 = Wait (ms)(milliseconds to wait=u32 20) -> ()  [unwired: 1 out]
                    n265 = Concatenate Strings("#0600FF" ("string"), "\r\n") -> (w593:string)
                    n266 = VISA Write(VISA resource name=w589, write buffer=w593, error in (no error)=w588) -> (VISA resource name out=w586:refnum<visa-resource-name>, error out=w587:errorcluster)  [unwired: 1 out]
                  }
                }
                n267 = Wait (ms)(milliseconds to wait=u32 20) -> ()  [unwired: 1 out]
              }
            }
            n268 = local write "rele 0_4"(w546) -> ()
            n269 = local write "rele 1_4"(w546) -> ()
            n270 = local write "rele 2_4"(w546) -> ()
            n271 = local write "rele 3_4"(w546) -> ()
            n272 = local write "rele 4_4"(w546) -> ()
            n273 = local write "rele 5_4"(w546) -> ()
            n274 = local write "rele 6_4"(w546) -> ()
            n275 = local write "rele 7_4"(w546) -> ()
            n276 = local write "rele 0_5"(w546) -> ()
            n277 = local write "rele 1_5"(w546) -> ()
            n278 = local write "rele 2_5"(w546) -> ()
            n279 = local write "rele 3_5"(w546) -> ()
            n280 = local write "rele 4_5"(w546) -> ()
            n281 = local write "rele 5_5"(w546) -> ()
            n282 = local write "rele 6_5"(w546) -> ()
            n283 = local write "rele 7_5"(w546) -> ()
            n284 = local write "rele 0_6"(w546) -> ()
            n285 = local write "rele 1_6"(w546) -> ()
            n286 = local write "rele 2_6"(w546) -> ()
            n287 = local write "rele 3_6"(w546) -> ()
            n288 = local write "rele 4_6"(w546) -> ()
            n289 = local write "rele 5_6"(w546) -> ()
            n290 = local write "rele 6_6"(w546) -> ()
            n291 = local write "rele 7_6"(w546) -> ()
          }
        }
        n292 = VISA Clear(VISA resource name=w495, error in (no error)=w496) -> (VISA resource name out=w493:refnum<visa-resource-name>, error out=w494:errorcluster)
      }
      event "rele 0_5": Value Change {
        n293 = event-data() -> ("NewVal"=w599:bool)  [unwired: 1 in]
        n294 = call-poly "VISA Configure Serial Port"("VISA resource name"=w594) -> ("VISA resource name out"=w596:refnum<visa-resource-name>, "error out"=w595:errorcluster)  [unwired: 13 in]
        n295 = case shown="True" w599 {
          tunnel: [w606 w614] -> w601
          tunnel: [w605 w613] -> w600
          tunnel: w595 -> [w604 w612]
          tunnel: w596 -> [w603 w611]
          frame False {
            n296 = Wait (ms)(milliseconds to wait=u32 20) -> ()  [unwired: 1 out]
            n297 = Concatenate Strings("#051000" ("string"), "\r\n") -> (w609:string)
            n298 = VISA Write(VISA resource name=w603, write buffer=w609, error in (no error)=w604) -> (VISA resource name out=w606:refnum<visa-resource-name>, error out=w605:errorcluster)  [unwired: 1 out]
          }
          frame True {
            n299 = Wait (ms)(milliseconds to wait=u32 20) -> ()  [unwired: 1 out]
            n300 = Concatenate Strings("#051001" ("string"), "\r\n") -> (w617:string)
            n301 = VISA Write(VISA resource name=w611, write buffer=w617, error in (no error)=w612) -> (VISA resource name out=w614:refnum<visa-resource-name>, error out=w613:errorcluster)  [unwired: 1 out]
          }
        }
        n302 = VISA Clear(VISA resource name=w601, error in (no error)=w600) -> (VISA resource name out=w597:refnum<visa-resource-name>, error out=w598:errorcluster)
      }
      event "rele 1_5": Value Change {
        n303 = event-data() -> ("NewVal"=w623:bool)  [unwired: 1 in]
        n304 = call-poly "VISA Configure Serial Port"("VISA resource name"=w618) -> ("VISA resource name out"=w619:refnum<visa-resource-name>, "error out"=w620:errorcluster)  [unwired: 13 in]
        n305 = case shown="True" w623 {
          tunnel: [w630 w638] -> w625
          tunnel: [w629 w637] -> w624
          tunnel: w620 -> [w627 w635]
          tunnel: w619 -> [w626 w634]
          frame False {
            n306 = Wait (ms)(milliseconds to wait=u32 10) -> ()  [unwired: 1 out]
            n307 = Concatenate Strings("#051100" ("string"), "\r\n") -> (w633:string)
            n308 = VISA Write(VISA resource name=w626, write buffer=w633, error in (no error)=w627) -> (VISA resource name out=w629:refnum<visa-resource-name>, error out=w630:errorcluster)  [unwired: 1 out]
          }
          frame True {
            n309 = Wait (ms)(milliseconds to wait=u32 10) -> ()  [unwired: 1 out]
            n310 = Concatenate Strings("#051101" ("string"), "\r\n") -> (w641:string)
            n311 = VISA Write(VISA resource name=w634, write buffer=w641, error in (no error)=w635) -> (VISA resource name out=w637:refnum<visa-resource-name>, error out=w638:errorcluster)  [unwired: 1 out]
          }
        }
        n312 = VISA Clear(VISA resource name=w624, error in (no error)=w625) -> (VISA resource name out=w622:refnum<visa-resource-name>, error out=w621:errorcluster)
      }
      event "rele 2_5": Value Change {
        n313 = event-data() -> ("NewVal"=w647:bool)  [unwired: 1 in]
        n314 = call-poly "VISA Configure Serial Port"("VISA resource name"=w642) -> ("VISA resource name out"=w644:refnum<visa-resource-name>, "error out"=w643:errorcluster)  [unwired: 13 in]
        n315 = case shown="True" w647 {
          tunnel: [w652 w662] -> w649
          tunnel: [w651 w661] -> w648
          tunnel: w644 -> [w654 w660]
          tunnel: w643 -> [w653 w659]
          frame False {
            n316 = Wait (ms)(milliseconds to wait=u32 10) -> ()  [unwired: 1 out]
            n317 = Concatenate Strings("#051200" ("string"), "\r\n") -> (w657:string)
            n318 = VISA Write(VISA resource name=w654, write buffer=w657, error in (no error)=w653) -> (VISA resource name out=w651:refnum<visa-resource-name>, error out=w652:errorcluster)  [unwired: 1 out]
          }
          frame True {
            n319 = Wait (ms)(milliseconds to wait=u32 10) -> ()  [unwired: 1 out]
            n320 = Concatenate Strings("#051201" ("string"), "\r\n") -> (w665:string)
            n321 = VISA Write(VISA resource name=w660, write buffer=w665, error in (no error)=w659) -> (VISA resource name out=w661:refnum<visa-resource-name>, error out=w662:errorcluster)  [unwired: 1 out]
          }
        }
        n322 = VISA Clear(VISA resource name=w648, error in (no error)=w649) -> (VISA resource name out=w645:refnum<visa-resource-name>, error out=w646:errorcluster)
      }
      event "rele 3_5": Value Change {
        n323 = event-data() -> ("NewVal"=w671:bool)  [unwired: 1 in]
        n324 = call-poly "VISA Configure Serial Port"("VISA resource name"=w666) -> ("VISA resource name out"=w668:refnum<visa-resource-name>, "error out"=w667:errorcluster)  [unwired: 13 in]
        n325 = case shown="True" w671 {
          tunnel: w668 -> [w678 w686]
          tunnel: w667 -> [w677 w685]
          tunnel: [w676 w683] -> w672
          tunnel: [w675 w684] -> w673
          frame False {
            n326 = Wait (ms)(milliseconds to wait=u32 10) -> ()  [unwired: 1 out]
            n327 = Concatenate Strings("#051300" ("string"), "\r\n") -> (w681:string)
            n328 = VISA Write(VISA resource name=w678, write buffer=w681, error in (no error)=w677) -> (VISA resource name out=w675:refnum<visa-resource-name>, error out=w676:errorcluster)  [unwired: 1 out]
          }
          frame True {
            n329 = Wait (ms)(milliseconds to wait=u32 10) -> ()  [unwired: 1 out]
            n330 = Concatenate Strings("#051301" ("string"), "\r\n") -> (w689:string)
            n331 = VISA Write(VISA resource name=w686, write buffer=w689, error in (no error)=w685) -> (VISA resource name out=w684:refnum<visa-resource-name>, error out=w683:errorcluster)  [unwired: 1 out]
          }
        }
        n332 = VISA Clear(VISA resource name=w673, error in (no error)=w672) -> (VISA resource name out=w669:refnum<visa-resource-name>, error out=w670:errorcluster)
      }
      event "rele 4_5": Value Change {
        n333 = event-data() -> ("NewVal"=w695:bool)  [unwired: 1 in]
        n334 = call-poly "VISA Configure Serial Port"("VISA resource name"=w690) -> ("VISA resource name out"=w691:refnum<visa-resource-name>, "error out"=w692:errorcluster)  [unwired: 13 in]
        n335 = case shown="False" w695 {
          tunnel: [w700 w710] -> w697
          tunnel: [w699 w709] -> w696
          tunnel: w692 -> [w702 w708]
          tunnel: w691 -> [w701 w707]
          frame False {
            n336 = Wait (ms)(milliseconds to wait=u32 10) -> ()  [unwired: 1 out]
            n337 = Concatenate Strings("#051400" ("string"), "\r\n") -> (w705:string)
            n338 = VISA Write(VISA resource name=w701, write buffer=w705, error in (no error)=w702) -> (VISA resource name out=w699:refnum<visa-resource-name>, error out=w700:errorcluster)  [unwired: 1 out]
          }
          frame True {
            n339 = Wait (ms)(milliseconds to wait=u32 10) -> ()  [unwired: 1 out]
            n340 = Concatenate Strings("#051401" ("string"), "\r\n") -> (w713:string)
            n341 = VISA Write(VISA resource name=w707, write buffer=w713, error in (no error)=w708) -> (VISA resource name out=w709:refnum<visa-resource-name>, error out=w710:errorcluster)  [unwired: 1 out]
          }
        }
        n342 = VISA Clear(VISA resource name=w696, error in (no error)=w697) -> (VISA resource name out=w693:refnum<visa-resource-name>, error out=w694:errorcluster)
      }
      event "rele 5_5": Value Change {
        n343 = event-data() -> ("NewVal"=w717:bool)  [unwired: 1 in]
        n344 = call-poly "VISA Configure Serial Port"("VISA resource name"=w714) -> ("VISA resource name out"=w715:refnum<visa-resource-name>, "error out"=w716:errorcluster)  [unwired: 13 in]
        n345 = case shown="False" w717 {
          tunnel: [w725 w733] -> w721
          tunnel: [w724 w732] -> w720
          tunnel: w715 -> [w723 w730]
          tunnel: w716 -> [w722 w731]
          frame False {
            n346 = Wait (ms)(milliseconds to wait=u32 10) -> ()  [unwired: 1 out]
            n347 = Concatenate Strings("#051500" ("string"), "\r\n") -> (w729:string)
            n348 = VISA Write(VISA resource name=w723, write buffer=w729, error in (no error)=w722) -> (VISA resource name out=w724:refnum<visa-resource-name>, error out=w725:errorcluster)  [unwired: 1 out]
          }
          frame True {
            n349 = Wait (ms)(milliseconds to wait=u32 10) -> ()  [unwired: 1 out]
            n350 = Concatenate Strings("#051501" ("string"), "\r\n") -> (w737:string)
            n351 = VISA Write(VISA resource name=w730, write buffer=w737, error in (no error)=w731) -> (VISA resource name out=w732:refnum<visa-resource-name>, error out=w733:errorcluster)  [unwired: 1 out]
          }
        }
        n352 = VISA Clear(VISA resource name=w720, error in (no error)=w721) -> (VISA resource name out=w718:refnum<visa-resource-name>, error out=w719:errorcluster)
      }
      event "rele 6_5": Value Change {
        n353 = event-data() -> ("NewVal"=w743:bool)  [unwired: 1 in]
        n354 = call-poly "VISA Configure Serial Port"("VISA resource name"=w738) -> ("VISA resource name out"=w739:refnum<visa-resource-name>, "error out"=w740:errorcluster)  [unwired: 13 in]
        n355 = case shown="False" w743 {
          tunnel: [w750 w757] -> w744
          tunnel: [w749 w758] -> w745
          tunnel: w740 -> [w748 w756]
          tunnel: w739 -> [w747 w755]
          frame False {
            n356 = Wait (ms)(milliseconds to wait=u32 10) -> ()  [unwired: 1 out]
            n357 = Concatenate Strings("#051600" ("string"), "\r\n") -> (w753:string)
            n358 = VISA Write(VISA resource name=w747, write buffer=w753, error in (no error)=w748) -> (VISA resource name out=w749:refnum<visa-resource-name>, error out=w750:errorcluster)  [unwired: 1 out]
          }
          frame True {
            n359 = Wait (ms)(milliseconds to wait=u32 10) -> ()  [unwired: 1 out]
            n360 = Concatenate Strings("#051601" ("string"), "\r\n") -> (w761:string)
            n361 = VISA Write(VISA resource name=w755, write buffer=w761, error in (no error)=w756) -> (VISA resource name out=w758:refnum<visa-resource-name>, error out=w757:errorcluster)  [unwired: 1 out]
          }
        }
        n362 = VISA Clear(VISA resource name=w745, error in (no error)=w744) -> (VISA resource name out=w741:refnum<visa-resource-name>, error out=w742:errorcluster)
      }
      event "rele 7_5": Value Change {
        n363 = event-data() -> ("NewVal"=w767:bool)  [unwired: 1 in]
        n364 = call-poly "VISA Configure Serial Port"("VISA resource name"=w762) -> ("VISA resource name out"=w763:refnum<visa-resource-name>, "error out"=w764:errorcluster)  [unwired: 13 in]
        n365 = case shown="True" w767 {
          tunnel: w764 -> [w773 w778]
          tunnel: w763 -> [w772 w779]
          tunnel: [w771 w782] -> w768
          tunnel: [w770 w781] -> w769
          frame False {
            n366 = Wait (ms)(milliseconds to wait=u32 10) -> ()  [unwired: 1 out]
            n367 = Concatenate Strings("#051700" ("string"), "\r\n") -> (w777:string)
            n368 = VISA Write(VISA resource name=w772, write buffer=w777, error in (no error)=w773) -> (VISA resource name out=w770:refnum<visa-resource-name>, error out=w771:errorcluster)  [unwired: 1 out]
          }
          frame True {
            n369 = Wait (ms)(milliseconds to wait=u32 10) -> ()  [unwired: 1 out]
            n370 = Concatenate Strings("#051701" ("string"), "\r\n") -> (w785:string)
            n371 = VISA Write(VISA resource name=w779, write buffer=w785, error in (no error)=w778) -> (VISA resource name out=w781:refnum<visa-resource-name>, error out=w782:errorcluster)  [unwired: 1 out]
          }
        }
        n372 = VISA Clear(VISA resource name=w769, error in (no error)=w768) -> (VISA resource name out=w765:refnum<visa-resource-name>, error out=w766:errorcluster)
      }
      event "rele 0_6": Value Change {
        n373 = event-data() -> ("NewVal"=w791:bool)  [unwired: 1 in]
        n374 = call-poly "VISA Configure Serial Port"("VISA resource name"=w788) -> ("VISA resource name out"=w786:refnum<visa-resource-name>, "error out"=w787:errorcluster)  [unwired: 13 in]
        n375 = case shown="False" w791 {
          tunnel: [w798 w806] -> w792
          tunnel: [w797 w805] -> w793
          tunnel: w787 -> [w796 w804]
          tunnel: w786 -> [w794 w802]
          frame False {
            n376 = Wait (ms)(milliseconds to wait=u32 10) -> ()  [unwired: 1 out]
            n377 = Concatenate Strings("#061000" ("string"), "\r\n") -> (w801:string)
            n378 = VISA Write(VISA resource name=w794, write buffer=w801, error in (no error)=w796) -> (VISA resource name out=w798:refnum<visa-resource-name>, error out=w797:errorcluster)  [unwired: 1 out]
          }
          frame True {
            n379 = Wait (ms)(milliseconds to wait=u32 10) -> ()  [unwired: 1 out]
            n380 = Concatenate Strings("#061001" ("string"), "\r\n") -> (w809:string)
            n381 = VISA Write(VISA resource name=w802, write buffer=w809, error in (no error)=w804) -> (VISA resource name out=w806:refnum<visa-resource-name>, error out=w805:errorcluster)  [unwired: 1 out]
          }
        }
        n382 = VISA Clear(VISA resource name=w792, error in (no error)=w793) -> (VISA resource name out=w789:refnum<visa-resource-name>, error out=w790:errorcluster)
      }
      event "rele 1_6": Value Change {
        n383 = event-data() -> ("NewVal"=w815:bool)  [unwired: 1 in]
        n384 = call-poly "VISA Configure Serial Port"("VISA resource name"=w810) -> ("VISA resource name out"=w812:refnum<visa-resource-name>, "error out"=w811:errorcluster)  [unwired: 13 in]
        n385 = case shown="True" w815 {
          tunnel: [w822 w830] -> w817
          tunnel: [w821 w829] -> w816
          tunnel: w811 -> [w819 w827]
          tunnel: w812 -> [w818 w826]
          frame False {
            n386 = Wait (ms)(milliseconds to wait=u32 10) -> ()  [unwired: 1 out]
            n387 = Concatenate Strings("#061100" ("string"), "\r\n") -> (w825:string)
            n388 = VISA Write(VISA resource name=w818, write buffer=w825, error in (no error)=w819) -> (VISA resource name out=w821:refnum<visa-resource-name>, error out=w822:errorcluster)  [unwired: 1 out]
          }
          frame True {
            n389 = Wait (ms)(milliseconds to wait=u32 10) -> ()  [unwired: 1 out]
            n390 = Concatenate Strings("#061101" ("string"), "\r\n") -> (w833:string)
            n391 = VISA Write(VISA resource name=w826, write buffer=w833, error in (no error)=w827) -> (VISA resource name out=w829:refnum<visa-resource-name>, error out=w830:errorcluster)  [unwired: 1 out]
          }
        }
        n392 = VISA Clear(VISA resource name=w816, error in (no error)=w817) -> (VISA resource name out=w813:refnum<visa-resource-name>, error out=w814:errorcluster)
      }
      event "rele 2_6": Value Change {
        n393 = event-data() -> ("NewVal"=w839:bool)  [unwired: 1 in]
        n394 = call-poly "VISA Configure Serial Port"("VISA resource name"=w835) -> ("VISA resource name out"=w836:refnum<visa-resource-name>, "error out"=w834:errorcluster)  [unwired: 13 in]
        n395 = case shown="True" w839 {
          tunnel: [w844 w854] -> w840
          tunnel: [w843 w853] -> w841
          tunnel: w836 -> [w846 w852]
          tunnel: w834 -> [w845 w851]
          frame False {
            n396 = Wait (ms)(milliseconds to wait=u32 10) -> ()  [unwired: 1 out]
            n397 = Concatenate Strings("#061200" ("string"), "\r\n") -> (w849:string)
            n398 = VISA Write(VISA resource name=w846, write buffer=w849, error in (no error)=w845) -> (VISA resource name out=w843:refnum<visa-resource-name>, error out=w844:errorcluster)  [unwired: 1 out]
          }
          frame True {
            n399 = Wait (ms)(milliseconds to wait=u32 10) -> ()  [unwired: 1 out]
            n400 = Concatenate Strings("#061201" ("string"), "\r\n") -> (w857:string)
            n401 = VISA Write(VISA resource name=w852, write buffer=w857, error in (no error)=w851) -> (VISA resource name out=w853:refnum<visa-resource-name>, error out=w854:errorcluster)  [unwired: 1 out]
          }
        }
        n402 = VISA Clear(VISA resource name=w841, error in (no error)=w840) -> (VISA resource name out=w837:refnum<visa-resource-name>, error out=w838:errorcluster)
      }
      event "rele 3_6": Value Change {
        n403 = event-data() -> ("NewVal"=w863:bool)  [unwired: 1 in]
        n404 = call-poly "VISA Configure Serial Port"("VISA resource name"=w858) -> ("VISA resource name out"=w860:refnum<visa-resource-name>, "error out"=w859:errorcluster)  [unwired: 13 in]
        n405 = case shown="True" w863 {
          tunnel: w860 -> [w870 w878]
          tunnel: w859 -> [w869 w877]
          tunnel: [w868 w875] -> w864
          tunnel: [w867 w876] -> w865
          frame False {
            n406 = Wait (ms)(milliseconds to wait=u32 10) -> ()  [unwired: 1 out]
            n407 = Concatenate Strings("#061300" ("string"), "\r\n") -> (w873:string)
            n408 = VISA Write(VISA resource name=w870, write buffer=w873, error in (no error)=w869) -> (VISA resource name out=w867:refnum<visa-resource-name>, error out=w868:errorcluster)  [unwired: 1 out]
          }
          frame True {
            n409 = Wait (ms)(milliseconds to wait=u32 10) -> ()  [unwired: 1 out]
            n410 = Concatenate Strings("#061301" ("string"), "\r\n") -> (w881:string)
            n411 = VISA Write(VISA resource name=w878, write buffer=w881, error in (no error)=w877) -> (VISA resource name out=w876:refnum<visa-resource-name>, error out=w875:errorcluster)  [unwired: 1 out]
          }
        }
        n412 = VISA Clear(VISA resource name=w865, error in (no error)=w864) -> (VISA resource name out=w861:refnum<visa-resource-name>, error out=w862:errorcluster)
      }
      event "rele 4_6": Value Change {
        n413 = event-data() -> ("NewVal"=w887:bool)  [unwired: 1 in]
        n414 = call-poly "VISA Configure Serial Port"("VISA resource name"=w882) -> ("VISA resource name out"=w884:refnum<visa-resource-name>, "error out"=w883:errorcluster)  [unwired: 13 in]
        n415 = case shown="False" w887 {
          tunnel: [w892 w902] -> w889
          tunnel: [w891 w901] -> w888
          tunnel: w883 -> [w894 w900]
          tunnel: w884 -> [w893 w899]
          frame False {
            n416 = Wait (ms)(milliseconds to wait=u32 10) -> ()  [unwired: 1 out]
            n417 = Concatenate Strings("#061400" ("string"), "\r\n") -> (w897:string)
            n418 = VISA Write(VISA resource name=w893, write buffer=w897, error in (no error)=w894) -> (VISA resource name out=w891:refnum<visa-resource-name>, error out=w892:errorcluster)  [unwired: 1 out]
          }
          frame True {
            n419 = Wait (ms)(milliseconds to wait=u32 10) -> ()  [unwired: 1 out]
            n420 = Concatenate Strings("#061401" ("string"), "\r\n") -> (w905:string)
            n421 = VISA Write(VISA resource name=w899, write buffer=w905, error in (no error)=w900) -> (VISA resource name out=w901:refnum<visa-resource-name>, error out=w902:errorcluster)  [unwired: 1 out]
          }
        }
        n422 = VISA Clear(VISA resource name=w888, error in (no error)=w889) -> (VISA resource name out=w885:refnum<visa-resource-name>, error out=w886:errorcluster)
      }
      event "rele 5_6": Value Change {
        n423 = event-data() -> ("NewVal"=w911:bool)  [unwired: 1 in]
        n424 = call-poly "VISA Configure Serial Port"("VISA resource name"=w906) -> ("VISA resource name out"=w908:refnum<visa-resource-name>, "error out"=w907:errorcluster)  [unwired: 13 in]
        n425 = case shown="False" w911 {
          tunnel: [w917 w925] -> w913
          tunnel: [w916 w924] -> w912
          tunnel: w908 -> [w915 w922]
          tunnel: w907 -> [w914 w923]
          frame False {
            n426 = Wait (ms)(milliseconds to wait=u32 10) -> ()  [unwired: 1 out]
            n427 = Concatenate Strings("#061500" ("string"), "\r\n") -> (w921:string)
            n428 = VISA Write(VISA resource name=w915, write buffer=w921, error in (no error)=w914) -> (VISA resource name out=w916:refnum<visa-resource-name>, error out=w917:errorcluster)  [unwired: 1 out]
          }
          frame True {
            n429 = Wait (ms)(milliseconds to wait=u32 10) -> ()  [unwired: 1 out]
            n430 = Concatenate Strings("#061501" ("string"), "\r\n") -> (w929:string)
            n431 = VISA Write(VISA resource name=w922, write buffer=w929, error in (no error)=w923) -> (VISA resource name out=w924:refnum<visa-resource-name>, error out=w925:errorcluster)  [unwired: 1 out]
          }
        }
        n432 = VISA Clear(VISA resource name=w912, error in (no error)=w913) -> (VISA resource name out=w909:refnum<visa-resource-name>, error out=w910:errorcluster)
      }
      event "rele 6_6": Value Change {
        n433 = event-data() -> ("NewVal"=w935:bool)  [unwired: 1 in]
        n434 = call-poly "VISA Configure Serial Port"("VISA resource name"=w930) -> ("VISA resource name out"=w932:refnum<visa-resource-name>, "error out"=w931:errorcluster)  [unwired: 13 in]
        n435 = case shown="False" w935 {
          tunnel: [w942 w949] -> w936
          tunnel: [w941 w950] -> w937
          tunnel: w931 -> [w940 w948]
          tunnel: w932 -> [w939 w947]
          frame False {
            n436 = Wait (ms)(milliseconds to wait=u32 10) -> ()  [unwired: 1 out]
            n437 = Concatenate Strings("#061600" ("string"), "\r\n") -> (w945:string)
            n438 = VISA Write(VISA resource name=w939, write buffer=w945, error in (no error)=w940) -> (VISA resource name out=w941:refnum<visa-resource-name>, error out=w942:errorcluster)  [unwired: 1 out]
          }
          frame True {
            n439 = Wait (ms)(milliseconds to wait=u32 10) -> ()  [unwired: 1 out]
            n440 = Concatenate Strings("#061601" ("string"), "\r\n") -> (w953:string)
            n441 = VISA Write(VISA resource name=w947, write buffer=w953, error in (no error)=w948) -> (VISA resource name out=w950:refnum<visa-resource-name>, error out=w949:errorcluster)  [unwired: 1 out]
          }
        }
        n442 = VISA Clear(VISA resource name=w937, error in (no error)=w936) -> (VISA resource name out=w933:refnum<visa-resource-name>, error out=w934:errorcluster)
      }
      event "rele 7_6": Value Change {
        n443 = event-data() -> ("NewVal"=w959:bool)  [unwired: 1 in]
        n444 = call-poly "VISA Configure Serial Port"("VISA resource name"=w954) -> ("VISA resource name out"=w956:refnum<visa-resource-name>, "error out"=w955:errorcluster)  [unwired: 13 in]
        n445 = case shown="False" w959 {
          tunnel: w955 -> [w965 w970]
          tunnel: w956 -> [w964 w971]
          tunnel: [w963 w974] -> w961
          tunnel: [w962 w973] -> w960
          frame False {
            n446 = Wait (ms)(milliseconds to wait=u32 10) -> ()  [unwired: 1 out]
            n447 = Concatenate Strings("#061700" ("string"), "\r\n") -> (w969:string)
            n448 = VISA Write(VISA resource name=w964, write buffer=w969, error in (no error)=w965) -> (VISA resource name out=w962:refnum<visa-resource-name>, error out=w963:errorcluster)  [unwired: 1 out]
          }
          frame True {
            n449 = Wait (ms)(milliseconds to wait=u32 10) -> ()  [unwired: 1 out]
            n450 = Concatenate Strings("#061701" ("string"), "\r\n") -> (w977:string)
            n451 = VISA Write(VISA resource name=w971, write buffer=w977, error in (no error)=w970) -> (VISA resource name out=w973:refnum<visa-resource-name>, error out=w974:errorcluster)  [unwired: 1 out]
          }
        }
        n452 = VISA Clear(VISA resource name=w960, error in (no error)=w961) -> (VISA resource name out=w957:refnum<visa-resource-name>, error out=w958:errorcluster)
      }
    }
    n453 = VISA Close(VISA resource name=w2, error in (no error)=w3) -> ()  [unwired: 1 out]
  }
